vi "manage time frame.vi"(6 "frame offset phase":dbl(slide)=0.0001 scale=0.0..100.0, 7 "time frame control":T2, 9 "frame step":dbl=0.002 format="%#_3p", 10 "frame inter":dbl=0.0001 format="%#_3p", 11 "frame":T1={"left"=0.0723, "right"=0.0727} {"right" format="%#_3p"; "left" format="%#_3p"}) -> (0 "Boolean":bool, 1 "frame step OUT":dbl=0.002 format="%#_3p", 2 "frame inter OUT":dbl=0.0001 format="%#_3p", 3 "frame out":T1={"left"=0.0723, "right"=0.0727} {"right" format="%#_3p"; "left" format="%#_3p"})   [LabVIEW 2021]
uses:
  manage time frame -- control.ctl
  time frame.ctl
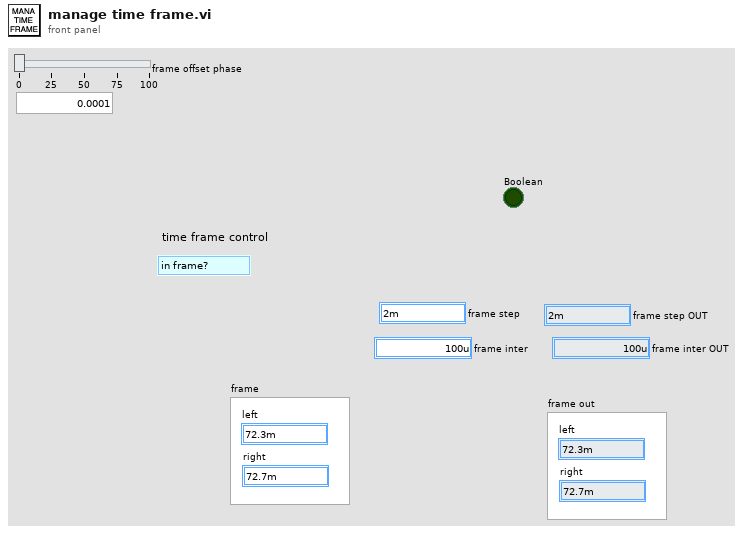
[diagram p1: front panel]
types:
  T1 = typedef "time frame.ctl" = cluster{"left":dbl, "right":dbl}
  T2 = typedef "manage time frame -- control.ctl" = enum16{"in frame?", "set frame", "next frame"}
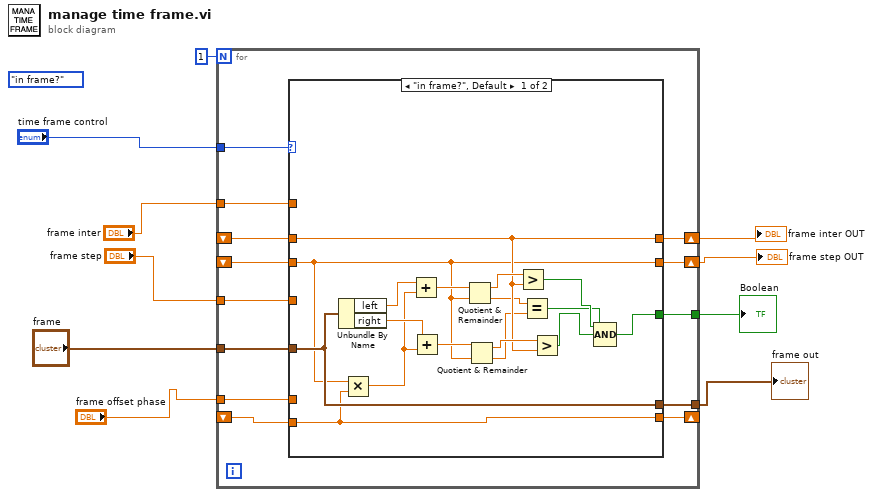
[diagram p0: block diagram]
diagram:
  (unwired) manage_time_frame_--_control."in frame?" ("time frame control")
  n1 = for {
    N: 1 -> [_]
    tunnel: "time frame control" -> [w23]
    tunnel: "frame inter" -> [w21]
    shift-right: [w22] -> w4
    shift-left: _ -> [w18]
    tunnel: "frame step" -> [w19]
    shift-right: [w20] -> w3
    shift-left: _ -> [w17]
    tunnel: "frame" -> [w16]
    tunnel: [w15] -> w5
    tunnel: [w14] -> w2
    shift-right: [w12] -> _
    shift-left: _ -> [w13]
    tunnel: "frame offset phase" -> [w11]
    n2 = case shown="\"in frame?\", Default" w23 {
      tunnel: [w38 w44] -> w22
      tunnel: w21 -> [_ w44]
      tunnel: [w25 w43] -> w20
      tunnel: w19 -> [_ w43]
      tunnel: w18 -> [w38 _]
      tunnel: w17 -> [w25 _]
      tunnel: w16 -> [w31 w42]
      tunnel: [w32 _] -> w15
      tunnel: [w31 w42] -> w14
      tunnel: w13 -> [w26 _]
      tunnel: [w26 w41] -> w12
      tunnel: w11 -> [_ w41]
      frame "in frame?", Default {
        n3 = Unbundle By Name(w31) -> ("left"=w30:dbl, "right"=w29:dbl)
        n4 = Multiply(x=w25, y=w26) -> (x*y=w24:dbl)
        n5 = Add(x=w30, y=w24) -> (x+y=w27:dbl)
        n6 = Add(x=w29, y=w24) -> (x+y=w28:dbl)
        n7 = Quotient & Remainder(x=w27, y=w25) -> (x-y*floor(x/y)=w40:dbl, floor(x/y)=w35:dbl)
        n8 = Quotient & Remainder(x=w28, y=w25) -> (x-y*floor(x/y)=w39:dbl, floor(x/y)=w34:dbl)
        n9 = Greater?(x=w40, y=w38) -> (0:w37:bool)
        n10 = Equal?(x=w35, y=w34) -> (x = y?=w33:bool)
        n11 = Greater?(x=w39, y=w38) -> (0:w36:bool)
        n12 = Compound Arithmetic op=AND(w37, w36, w33) -> (w32:bool)
      }
      frame "set frame" {
      }
    }
  }
  "Boolean" <- w5
  "frame step OUT" <- w3
  "frame inter OUT" <- w4
  "frame out" <- w2
